vi "action.vi"(0 "HB_PollingAgentVisitor in":refnum<class "HB_PollingAgentVisitor.lvclass">, 2 "HGF_Visitable":refnum<class "HGF_Visitable.lvclass">, 5 "error in (no error)":errorcluster) -> (14 "HB_PollingAgentVisitor out":refnum<class "HB_PollingAgentVisitor.lvclass">, 16 "dup HGF_Visitable":refnum<class "HGF_Visitable.lvclass">, 19 "error out":errorcluster)   [LabVIEW 2009, in "HB_PollingAgent.lvlib" / "HB_PollingAgentVisitor.lvclass"]
doc: "This is a dynamic dispatch VI that is called from Visitor.visit(). It will call member VIs of Visitable to perform the requested action which means: calling public methods of Visitable child class.\n\n<B>Hint:</B> This method is abstract and need to be implemented by child classes."
uses:
  HB_PollingAgentVisitor.lvclass
  lib.lib/HGF_LVC/HGF_BaseClasses/HGF_Visitable/HGF_Visitable.lvclass
  HB_PollingAgent/HB_PollingAgent.lvclass
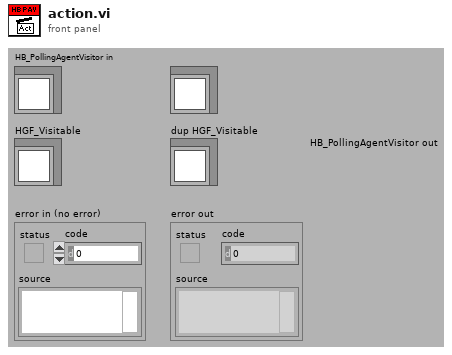
[diagram p1: front panel]
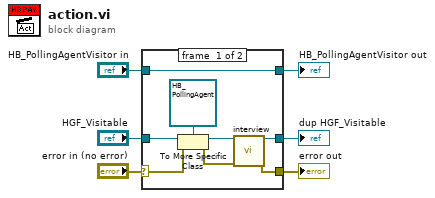
[diagram p0: block diagram]
diagram:
  n1 = case shown="No Error" "error in (no error)" {
    selector: "error in (no error)" -> [w8 w15]
    tunnel: "HGF_Visitable" -> [w14 w16]
    tunnel: [w10 w15] -> w5
    tunnel: "HB_PollingAgentVisitor in" -> [w7 w17]
    tunnel: [w7 w17] -> w3
    tunnel: [w9 w16] -> w2
    frame #0 {
      n2 = To More Specific Class(target class=refnum<class "HB_PollingAgent.lvclass"> refnum ("HB_PollingAgent.lvlib:HB_PollingAgent.lvclass"), reference=w14, error in=w8) -> (specific class reference=w12:refnum<class "HB_PollingAgent.lvclass">, error out=w11:errorcluster)
      n3 = call "interview.vi"("HB_PollingAgent in"=w12, "error in (no error)"=w11) -> ("HB_PollingAgent out"=w9:refnum<class "HB_PollingAgent.lvclass">, "error out"=w10:errorcluster)  [unwired: 12 in]
    }
    frame #1 {
    }
  }
  "error out" <- w5
  "HB_PollingAgentVisitor out" <- w3
  "dup HGF_Visitable" <- w2
